vi "Activity Light - Core.vi"(1 "Bool Refnum":refnum<vi>, 2 "Name":string="Activity Light") -> ()   [LabVIEW 2024, in "EQMF.lvlib" / "Status Utils.lvlib"]
uses:
  Status Utils.lvlib
  _Private/Activity Light Q Item.ctl
  _Private/Activity Light Color Types.ctl
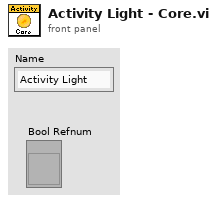
[diagram p1: front panel]
types:
  T1 = typedef "EQMF.lvlib/Status Utils.lvlib/Activity Light Q Item.ctl" = cluster{"Cmd":string, "Data":variant}
  T2 = typedef "EQMF.lvlib/Status Utils.lvlib/Activity Light Color Types.ctl" = enum16{"OK (Green)", "Active (Yellow)", "Warning (Orange)", "Error (Red)", "Attention (Blue)", "Custom Color"}
  T3 = cluster{"Type":T2, "ON Color":u32, "OFF Color":u32}
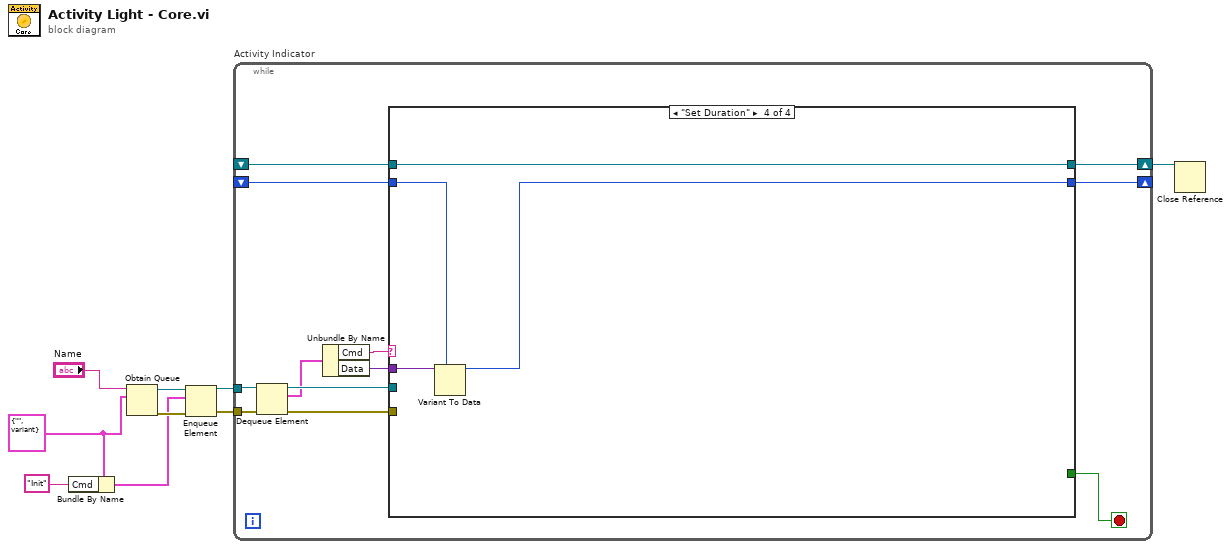
[diagram p0: block diagram]
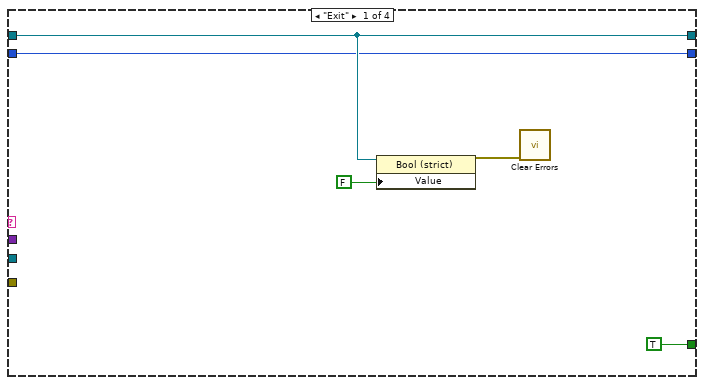
[diagram p2: hidden frame]
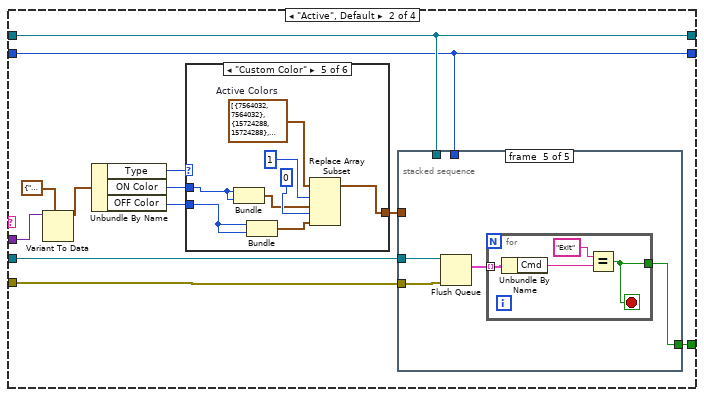
[diagram p3: hidden frame]
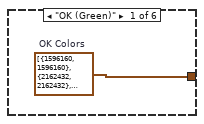
[diagram p4: hidden frame]
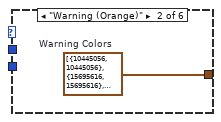
[diagram p5: hidden frame]
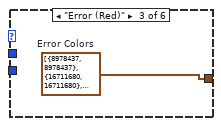
[diagram p6: hidden frame]
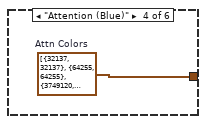
[diagram p7: hidden frame]
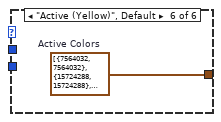
[diagram p8: hidden frame]
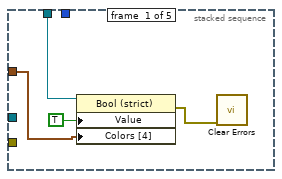
[diagram p9: hidden frame]
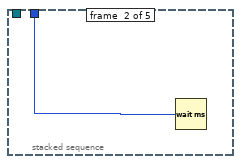
[diagram p10: hidden frame]
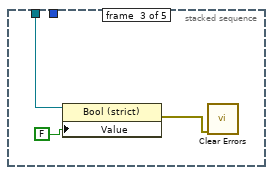
[diagram p11: hidden frame]
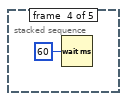
[diagram p12: hidden frame]
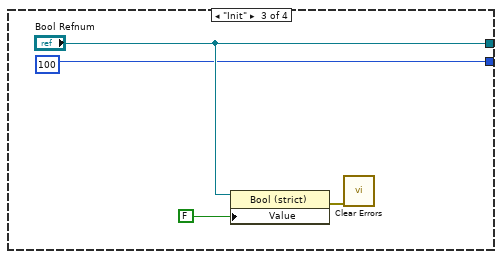
[diagram p13: hidden frame]
diagram:
  w2 = T1 {"Cmd"="", "Data"=variant} ("output cluster")
  n1 = Bundle By Name(cluster=w2, "Cmd"="Init") -> (w1:T1)
  n2 = Obtain Queue(name (unnamed)="Name", element data type=w2) -> (queue out=w8:refnum<queue>, error out=w5:errorcluster)  [unwired: 3 in, 1 out]
  n3 = Enqueue Element(queue=w8, element=w1, error in (no error)=w5) -> (queue out=w9:refnum<queue>, error out=w6:errorcluster)  [unwired: 1 in, 1 out]
  n4 = while "Activity Indicator" {
    tunnel: w9 -> [w21]
    shift-right: [w17] -> w4
    shift-left: _ -> [w16]
    tunnel: w6 -> [w15]
    shift-right: [w10] -> _
    shift-left: _ -> [w11]
    stop <- w20 stop-if-true
    n5 = Dequeue Element(queue=w21, error in (no error)=w15) -> (queue out=w19:refnum<queue>, element=w14:T1, error out=w18:errorcluster)  [unwired: 1 in, 1 out]
    n6 = Unbundle By Name(w14) -> ("Cmd"=w12:string, "Data"=w13:variant)
    n7 = case shown="\"Set Duration\"" w12 {
      tunnel: [TRUE w35 _ _] -> w20
      tunnel: w19 -> [_ w37 _ _]
      tunnel: w18 -> [_ w36 _ _]
      tunnel: [w25 w38 "Bool Refnum" w76] -> w17
      tunnel: w16 -> [w25 w38 _ w76]
      tunnel: w13 -> [_ w34 _ w75]
      tunnel: w11 -> [w22 w27 _ w74]
      tunnel: [w22 w27 u32 100 ("milliseconds to wait") w73] -> w10
      frame "Exit" {
        n8 = property class="Bool (strict)"(reference=w25, "Value"=FALSE) -> (error out=w24:errorcluster)  [unwired: 1 in, 1 out]
        n9 = call <vilib>:"Clear Errors.vi"("error in (no error)"=w24) -> ()  [unwired: 5 in, 2 out]
      }
      frame "Active", Default {
        n10 = Variant To Data(type=T3 {"Type"=enum."OK (Green)", "ON Color"=0, "OFF Color"=0} ("output cluster"), Variant=w34) -> (data=w33:T3)  [unwired: 1 in, 1 out]
        n11 = Unbundle By Name(w33) -> ("Type"=w31:T2, "ON Color"=w32:u32, "OFF Color"=w28:u32)
        n12 = case shown="\"Custom Color\"" w31 {
          tunnel: w32 -> [_ _ _ _ w43 _]
          tunnel: [w39 w40 w41 w42 w48 w51] -> w30
          tunnel: w28 -> [_ _ _ _ w47 _]
          frame "OK (Green)" {
            w39 = cluster{u32, u32}[] [{1596160, 1596160}, {2162432, 2162432}, {3749120, 3749120}, {6843904, 6843904}]  # OK Colors
          }
          frame "Warning (Orange)" {
            w40 = cluster{u32, u32}[] [{10445056, 10445056}, {15695616, 15695616}, {3749120, 3749120}, {6843904, 6843904}]  # Warning Colors
          }
          frame "Error (Red)" {
            w41 = cluster{u32, u32}[] [{8978437, 8978437}, {16711680, 16711680}, {3749120, 3749120}, {6843904, 6843904}]  # Error Colors
          }
          frame "Attention (Blue)" {
            w42 = cluster{u32, u32}[] [{32137, 32137}, {64255, 64255}, {3749120, 3749120}, {6843904, 6843904}]  # Attn Colors
          }
          frame "Custom Color" {
            w50 = cluster{u32, u32}[] [{7564032, 7564032}, {15724288, 15724288}, {3749120, 3749120}, {6843904, 6843904}]  # Active Colors
            n13 = Bundle("ON Color"=w43, "ON Color"=w43) -> (w45:cluster{"ON Color":u32, "ON Color":u32})  [unwired: 1 in]
            n14 = Bundle("OFF Color"=w47, "OFF Color"=w47) -> (w44:cluster{"OFF Color":u32, "OFF Color":u32})  [unwired: 1 in]
            n15 = Replace Array Subset(array=w50, new element #1=w45, index #1=1 ("index"), new element #2=w44, index #2=0 ("index")) -> (w48:cluster{u32, u32}[])
          }
          frame "Active (Yellow)", Default {
            w51 = cluster{u32, u32}[] [{7564032, 7564032}, {15724288, 15724288}, {3749120, 3749120}, {6843904, 6843904}]  # Active Colors
          }
        }
        n16 = stacked-sequence {
          tunnel: w38 -> [w54 _ w58 _ _]
          tunnel: w37 -> [_ _ _ _ w63]
          tunnel: w36 -> [_ _ _ _ w62]
          tunnel: [_ _ _ _ w61] -> w35
          tunnel: w30 -> [w52 _ _ _ _]
          tunnel: w27 -> [_ w56 _ _ _]
          frame #0 {
            n17 = property class="Bool (strict)"(reference=w54, "Value"=TRUE, "Colors [4]"=w52) -> (error out=w53:errorcluster)  [unwired: 1 in, 1 out]
            n18 = call <vilib>:"Clear Errors.vi"("error in (no error)"=w53) -> ()  [unwired: 5 in, 2 out]
          }
          frame #1 {
            n19 = Wait (ms)(milliseconds to wait=w56) -> ()  [unwired: 1 out]
          }
          frame #2 {
            n20 = property class="Bool (strict)"(reference=w58, "Value"=FALSE) -> (error out=w57:errorcluster)  [unwired: 1 in, 1 out]
            n21 = call <vilib>:"Clear Errors.vi"("error in (no error)"=w57) -> ()  [unwired: 5 in, 2 out]
          }
          frame #3 {
            n22 = Wait (ms)(milliseconds to wait=u32 60) -> ()  [unwired: 1 out]
          }
          frame #4 {
            n23 = Flush Queue(queue=w63, error in (no error)=w62) -> (remaining elements=w64:T1[])  [unwired: 2 out]
            n24 = for {
              tunnel: w64 -> [w66] mode=indexing
              tunnel: [w67] -> w61
              stop <- w67 stop-if-true
              n25 = Unbundle By Name(w66) -> ("Cmd"=w65:string)
              n26 = Equal?(x="Exit", y=w65) -> (x = y?=w67:bool)
            }
          }
        }
      }
      frame "Init" {
        n27 = property class="Bool (strict)"(reference="Bool Refnum", "Value"=FALSE) -> (error out=w71:errorcluster)  [unwired: 1 in, 1 out]
        n28 = call <vilib>:"Clear Errors.vi"("error in (no error)"=w71) -> ()  [unwired: 5 in, 2 out]
      }
      frame "Set Duration" {
        n29 = Variant To Data(type=w74, Variant=w75) -> (data=w73:u32)  [unwired: 1 in, 1 out]
      }
    }
  }
  n30 = Close Reference(reference=w4) -> ()  [unwired: 1 in, 1 out]
